vi "Main.vi"(11 "Module Admin":refnum<class "Delacor_lib_QMH_Cloneable Module Admin.lvclass">) -> ()   [LabVIEW 2016, in "Data Analysis.lvlib"]
doc: "This template is based off of the Queued Message Handler design pattern and the Queued Message Handler project template that ships with LabVIEW.\n\nThe main difference is that the queue is private to this module and communication between modules is performed via Broadcast and Request events.\n\nRequest events are wrapped in public API methods and are handled in the Event Handling Loop (EHL) of this VI. Any module can register for Broadcast events sent by this module. The EHL generates messages based on user interface actions.\n\nThe Message Handling Loop (MHL) processes messages generated by the EHL, or by other messages. The messages are string values, so new messages can be added easily to the Message Cases case structure in the MHL. Each message cluster can also provide an optional value for Message Data, which is a variant that can be converted to whatever message-specific data is required.\n_____\nBased on DQMH Project Template 6.1.0.94."
uses:
  Data Analysis.lvlib
  <vilib>/Delacor/Delacor QMH/Libraries/Cloneable Module Admin_class/Delacor_lib_QMH_Cloneable Module Admin.lvclass
  C:/Program Files (x86)/National Instruments/LabVIEW 2016/vi.lib/Delacor/Delacor QMH/Libraries/Module Admin_class/Delacor_lib_QMH_Module Admin.lvclass
  <vilib>/Delacor/Delacor QMH/Libraries/Cloneable Module Admin_class/Delacor_lib_QMH_Cloneable Module Admin.lvclass/Delacor_lib_QMH_Cloneable Module Admin.ctl
  Module Data--cluster.ctl
  <vilib>/Delacor/Delacor QMH/Libraries/Message Queue_class/Delacor_lib_QMH_Message Queue.lvclass/Delacor_lib_QMH_Message Queue.ctl
  Stop Argument--cluster.ctl
  REQ Initialize Selector Argument--cluster.ctl
  REQ Start Acq Argument--cluster.ctl
  REQ Signal Selection Argument--cluster.ctl
  REQ Stop Acq Argument--cluster.ctl
  <vilib>/Utility/miscctls.llb/LVPointTypeDef.ctl
  <vilib>/Delacor/Delacor QMH/Libraries/Module Admin_class/Delacor_lib_QMH_Module Admin.lvclass/Delacor_lib_QMH_Module Admin.ctl
  <vilib>/Delacor/Delacor QMH/Libraries/Cloneable Module Admin_class/Delacor_lib_QMH_Get Module ID.vi
  <vilib>/Delacor/Delacor QMH/Libraries/Message Queue_class/Delacor_lib_QMH_Enqueue Message (Single).vi
  Support Libraries/Current Value Table/DataTypes/Array of Double_Read.vi
  Support Libraries/Current Value Table/DataTypes/Double_Read.vi
  Support Libraries/Current Value Table/DataTypes/Single_Read.vi
  Support Libraries/Current Value Table/DataTypes/Boolean_Read.vi
  <vilib>/Delacor/Delacor QMH/Libraries/Module Admin_class/Delacor_lib_QMH_Get External Launch.vi
  Support Libraries/Current Value Table/Type to Enum.vi
  Support Libraries/Current Value Table/DataTypes/Array of Double_Type To Enum.vi
  Support Libraries/Current Value Table/DataTypes/Double_Type To Enum.vi
  Support Libraries/Current Value Table/DataTypes/Single_Type To Enum.vi
  Support Libraries/Current Value Table/DataTypes/Boolean_Type To Enum.vi
  <vilib>/Utility/error.llb/Error Cluster From Error Code.vi
  Support Libraries/Current Value Table/FGVs/Tag Memory.vi
  Support Libraries/Current Value Table/FGVs/CVT Globals.vi
  Support Libraries/Current Value Table/Memory Block.vi
  Support Libraries/Current Value Table/DataTypes/Array of Double_Memory Block.vi
  Support Libraries/Current Value Table/DataTypes/Double_Memory Block.vi
  Support Libraries/Current Value Table/DataTypes/Single_Memory Block.vi
  Support Libraries/Current Value Table/DataTypes/Boolean_Memory Block.vi
  <vilib>/ErrorRing/Error Ring.xnode
  <vilib>/Delacor/Delacor QMH/Libraries/Message Queue_class/Delacor_lib_QMH_Message Queue.lvclass
  User Interface/User Interface.lvlib
  Error Log/Error Log.lvlib
  Support Libraries/Current Value Table/Current Value Table.lvlib
panel:
  in  "Select Module":i32(ring)=-1 items=["All"=-1]
  in  "error in (no error)":errorcluster
  in  "Signal Selection":string[](tree)
  in  "Stop Button":bool
  in  "Start Button":bool
  out "Time":string="Sat  8/3/2019  8:10:44 PM"
  in  "Exit":bool
  out "Analog Data":dbl[][](graph)
  out "error out":errorcluster
  out "Status":string
  in  "Simulate EHL Error":bool
  in  "Simulate MHL Error":bool
  # "Other QMH Modules communicate with this Module via its Public API (wrappers for its Request Events).\n\nThis Module communicates with other Modules via its Broadcast Events.\nAny module that wants to get these messages, just registers for this module's Broadcast events."
  # "This template is for the Delacor Modified Queued Message Handler design pattern.\n\nSee the block diagram for more information on how to use this template."
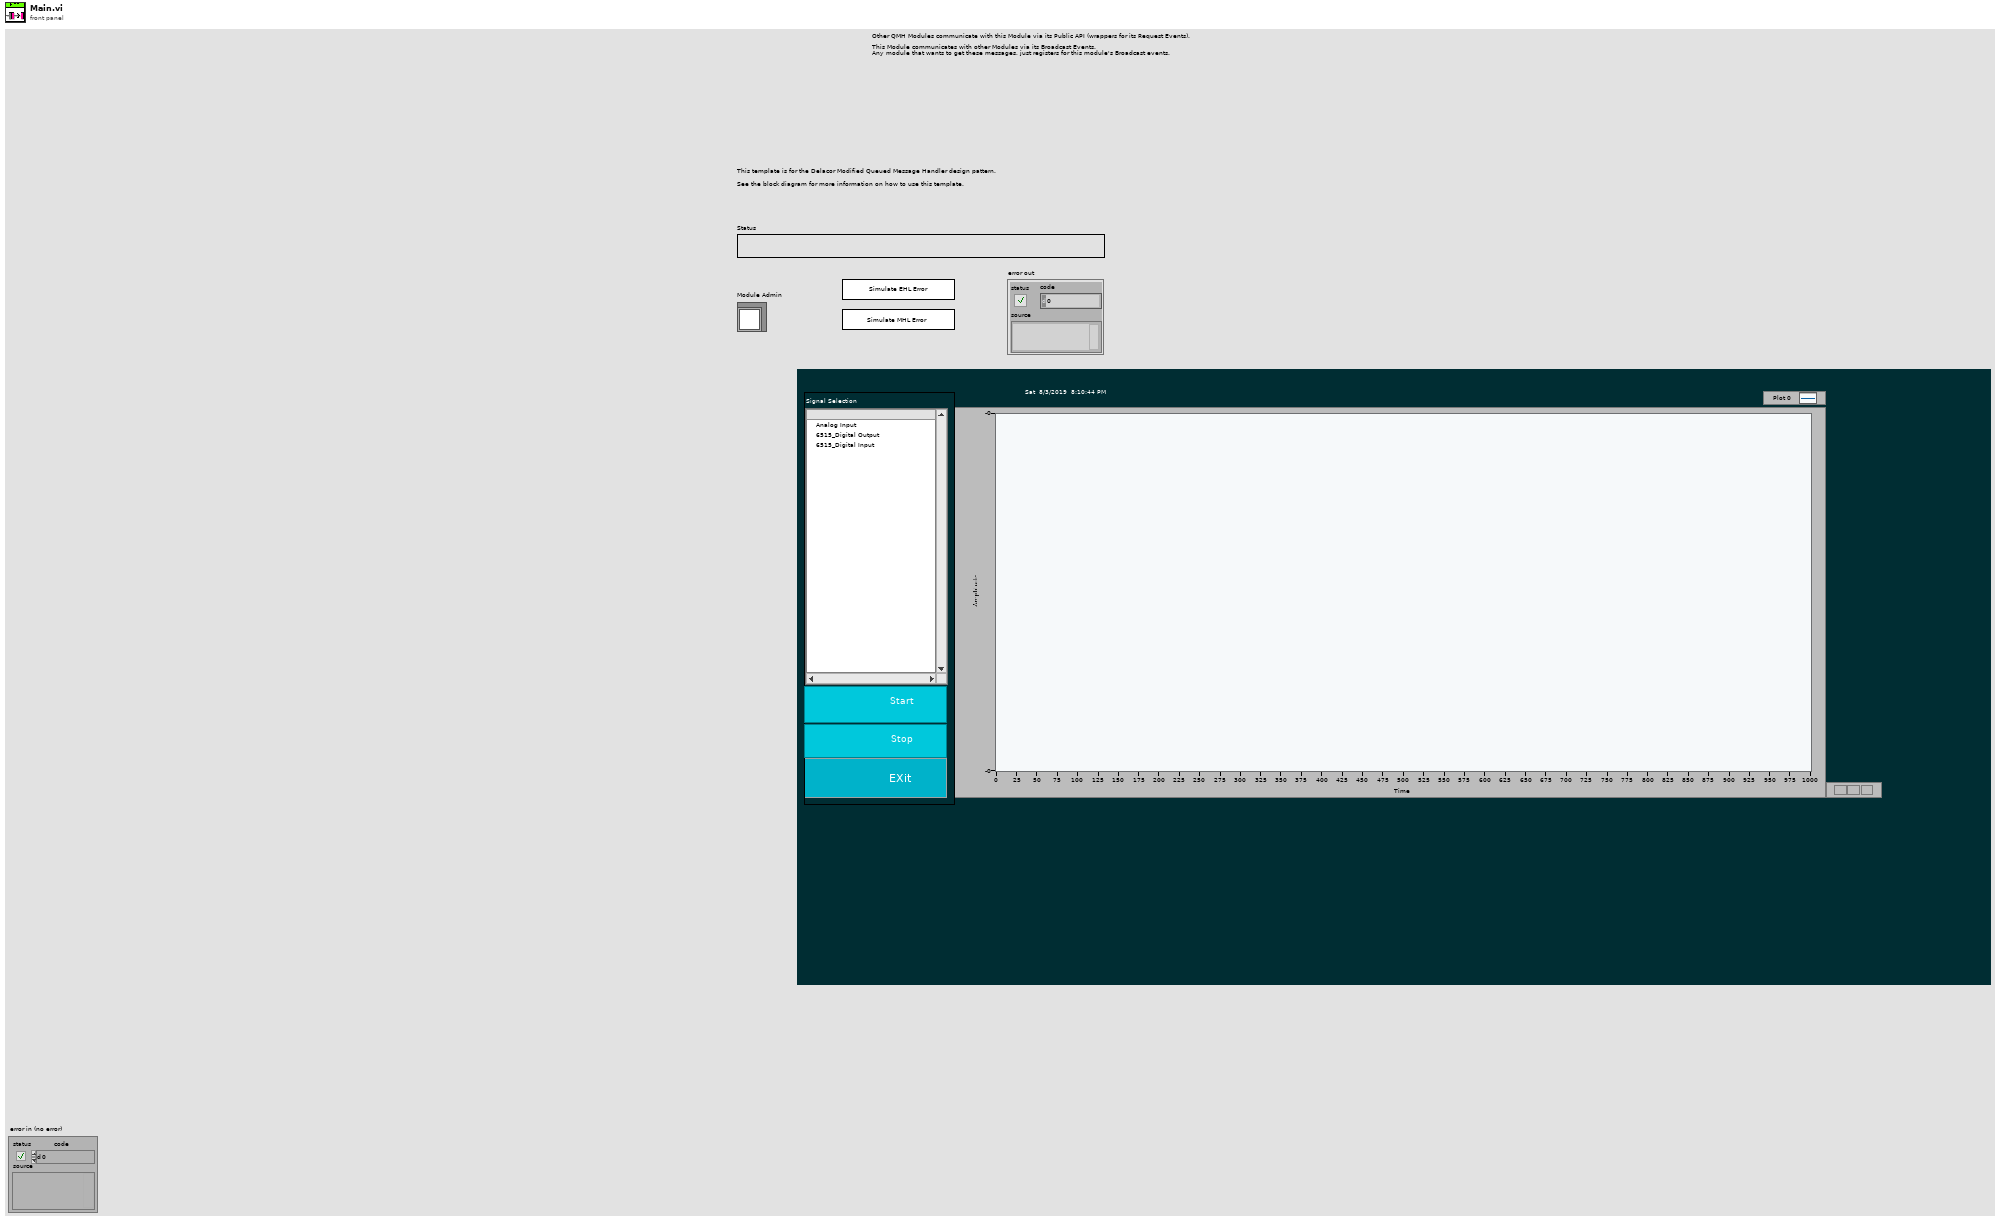
[diagram p1: front panel]
types:
  T1 = typedef "Data Analysis.lvlib/Request Events--cluster.ctl" = cluster{"Stop Module":refnum<user-event>, "Show Panel":refnum<user-event>, "Hide Panel":refnum<user-event>, "Show Diagram":refnum<user-event>, "Get Module Execution Status":refnum<user-event>, "REQ Initialize Selector":refnum<user-event>, "REQ Wakeup_help_loop":refnum<user-event>, "REQ Start Acq":refnum<user-event>, "REQ Signal Selection":refnum<user-event>, "REQ Stop Acq":refnum<user-event>}
  T2 = enum32{"invalid lock state", "Not Locked", "Locked (No Password)", "Password-protected"}
  T3 = typedef "Data Analysis.lvlib/Stop Argument--cluster.ctl" = cluster{"Module ID":i32, "Origin":string, "Exit via Stop Module Req?":bool, "Wait for Module to stop?":bool}
  T4 = typedef "Data Analysis.lvlib/REQ Initialize Selector Argument--cluster.ctl" = cluster{"Module ID":i32, "Boolean":bool}
  T5 = typedef "Data Analysis.lvlib/REQ Start Acq Argument--cluster.ctl" = cluster{"Module ID":i32, "Boolean":bool}
  T6 = typedef "Data Analysis.lvlib/REQ Signal Selection Argument--cluster.ctl" = cluster{"Module ID":i32, "Signal Selection":string[]}
  T7 = typedef "Data Analysis.lvlib/REQ Stop Acq Argument--cluster.ctl" = cluster{"Module ID":i32, "Boolean":bool}
  T8 = typedef "LVPointTypeDef.ctl" = cluster{"Horizontal":i16, "Vertical":i16}
  T9 = enum32{"Invalid", "Standard", "Closed", "Hidden", "Minimized", "Maximized"}
  T10 = typedef "Data Analysis.lvlib/Module Data--cluster.ctl" = cluster{"Status":string, "Signal Selecton":refnum<vi>, "Active Signal":string[], "Module ID":i32}
  T11 = typedef "CVT.lvlib/Current Value Table.lvlib/Data Types.ctl" = enum16{"Double", "Single", "I64", "I32", "I16", "I8", "U64", "U32", "U16", "U8", "String", "Boolean", "Array of U8", "Array of U16", "Array of U32", "Array of U64", "Array of I64", "Array of I32", "Array of I16", "Array of I8", "Array of Double", "Array of Single", "Array of Boolean", "Array of String"}
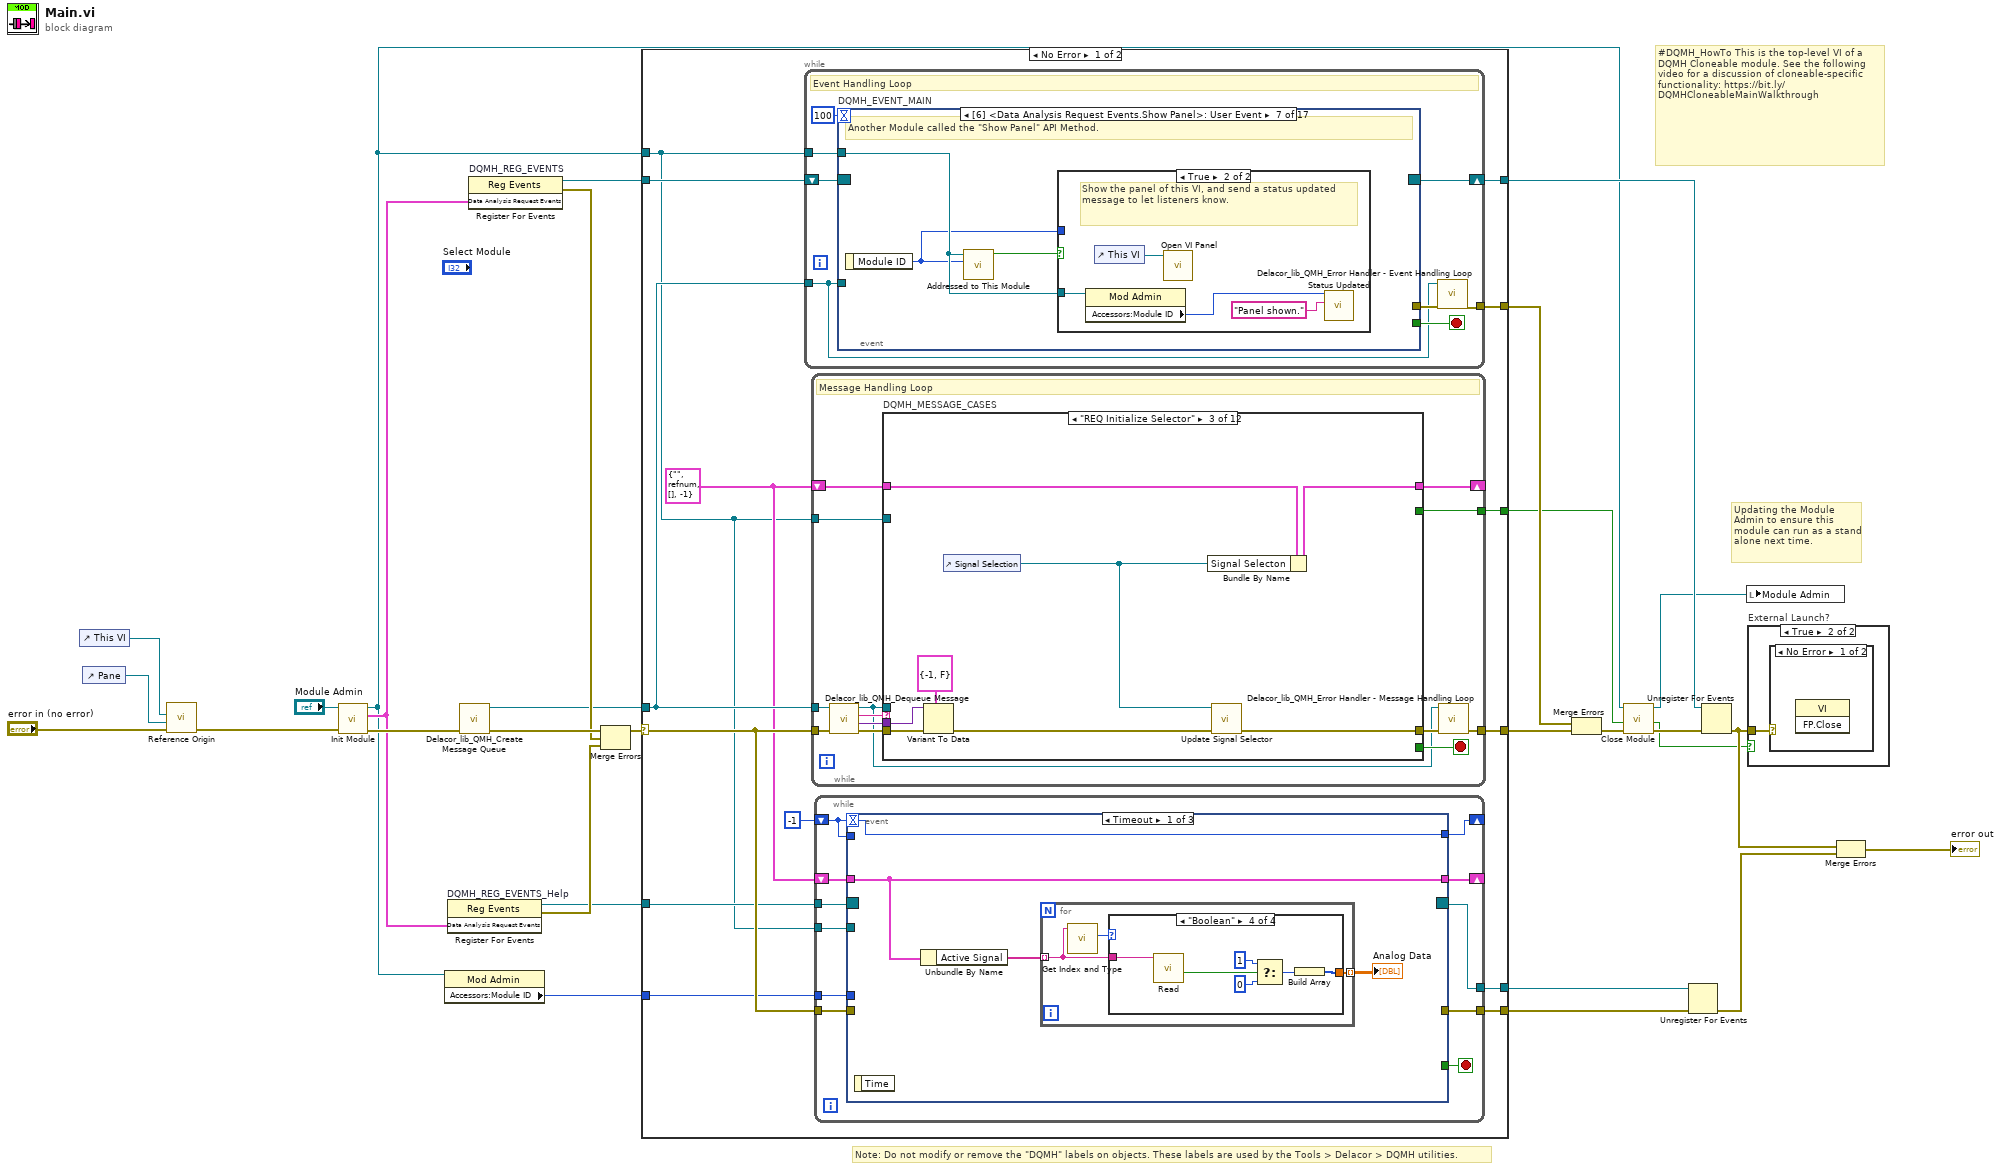
[diagram p0: block diagram]
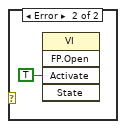
[diagram p3: hidden frame]
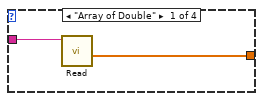
[diagram p4: hidden frame]
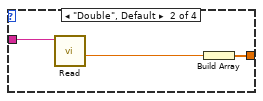
[diagram p5: hidden frame]
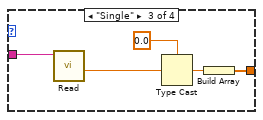
[diagram p6: hidden frame]
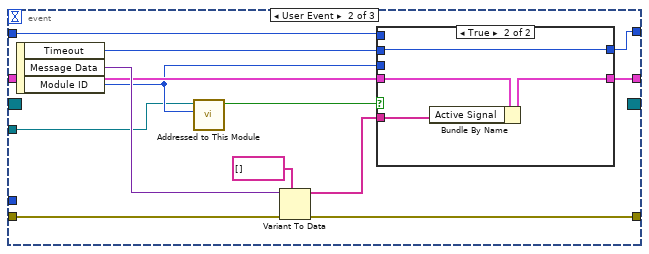
[diagram p7: hidden frame]
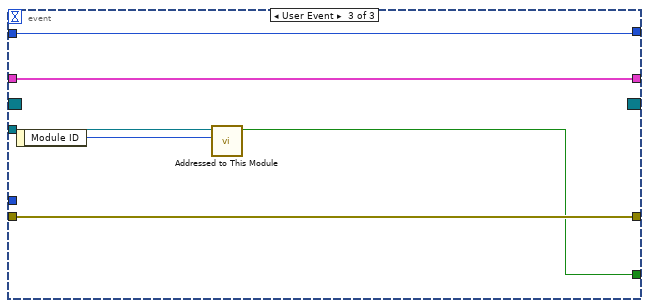
[diagram p9: hidden frame]
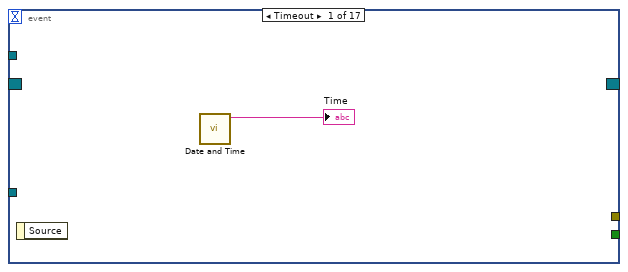
[diagram p10: hidden frame]
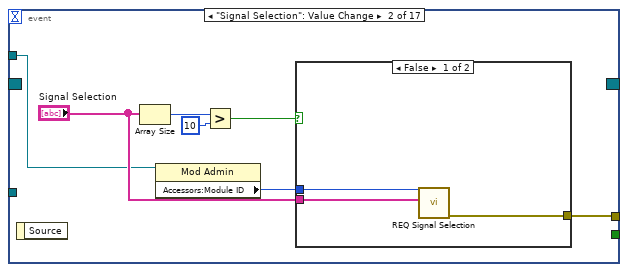
[diagram p11: hidden frame]
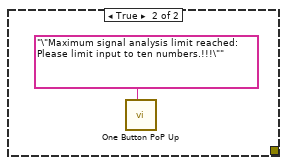
[diagram p12: hidden frame]
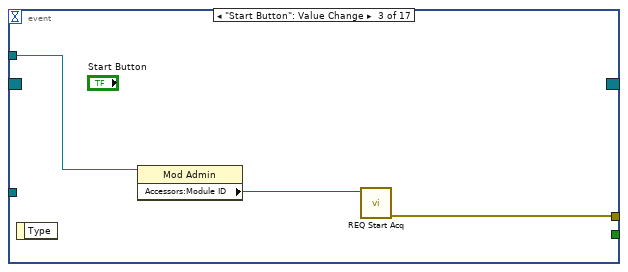
[diagram p13: hidden frame]
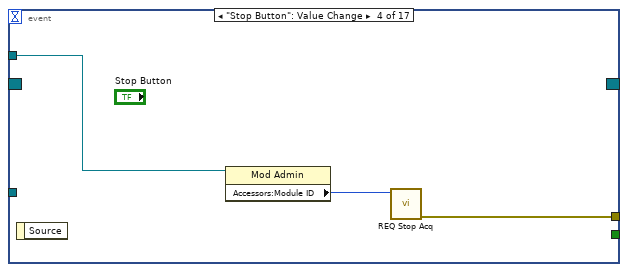
[diagram p14: hidden frame]
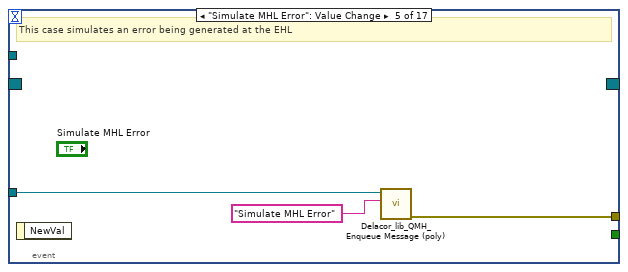
[diagram p15: hidden frame]
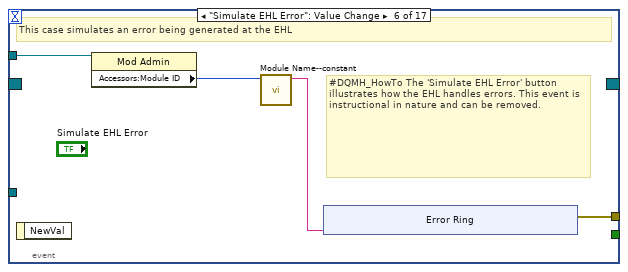
[diagram p16: hidden frame]
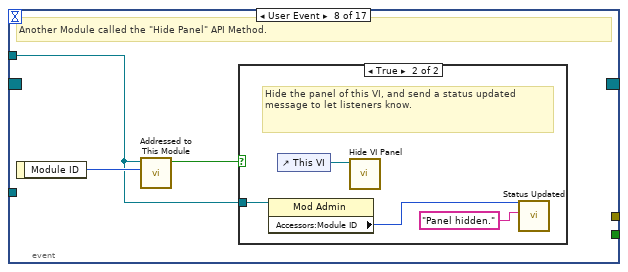
[diagram p18: hidden frame]
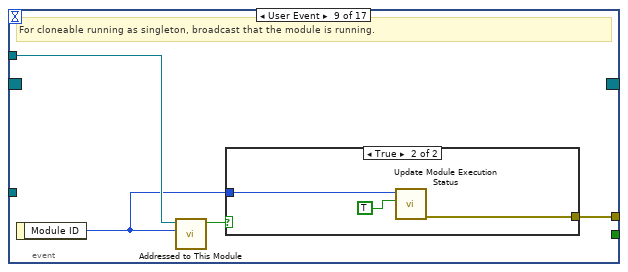
[diagram p20: hidden frame]
diagram:
  # "#DQMH_HowTo This is the top-level VI of a DQMH Cloneable module. See the following video for a discussion of cloneable-specific functionality: https://bit.ly/DQMHCloneableMainWalkthrough"
  # "Note: Do not modify or remove the \"DQMH\" labels on objects. These labels are used by the Tools > Delacor > DQMH utilities."
  # "Updating the Module Admin to ensure this module can run as a stand alone next time."
  n1 = control-ref of="This VI"() -> (w2:refnum<vi>)
  n2 = control-ref of="Pane"() -> (w1:refnum<vi>)
  n3 = call "Reference Origin.vi"("error in (no error)"="error in (no error)", "Pane"=w1, "This VI"=w2) -> ("error out"=w3:errorcluster)  [unwired: 8 in]
  n4 = call "Init Module.vi"("error in"=w3, "Cloneable Module Admin in"="Module Admin") -> ("error out"=w26:errorcluster, "Data Analysis Request Events"=w12:T1, "Cloneable Module Admin out"=w5:refnum<class "Delacor_lib_QMH_Cloneable Module Admin.lvclass">)  [unwired: 7 in]
  n5 = property class="Mod Admin"(reference=w5) -> ("Accessors:Module ID"=w4:i32)  [unwired: 1 in, 2 out]
  n6 = register-events "DQMH_REG_EVENTS_Help"(w12) -> (reference out=w10:refnum<event-registration>, error out=w11:errorcluster)  [unwired: 2 in]
  n7 = call <vilib>:"Delacor_lib_QMH_Create Message Queue.vi"("error in"=w26) -> ("error out"=w23:errorcluster, "Message Queue"=w18:refnum<class "Delacor_lib_QMH_Message Queue.lvclass">)  [unwired: 9 in]
  n8 = register-events "DQMH_REG_EVENTS"(w12) -> (reference out=w19:refnum<event-registration>, error out=w21:errorcluster)  [unwired: 2 in]
  n9 = Merge Errors(w23, w21, w11) -> (w22:errorcluster)
  n10 = case shown="No Error" w22 {
    selector: w22 -> [w37 w403]
    tunnel: [w43 w402] -> w27
    tunnel: [w41 w410] -> w20
    tunnel: w19 -> [w40 w410]
    tunnel: w18 -> [w39 w401]
    tunnel: [w42 _] -> w28
    tunnel: w5 -> [w30 w406]
    tunnel: [w38 _] -> w15
    tunnel: w10 -> [w36 w400]
    tunnel: [w35 _] -> w9
    tunnel: [w34 w400] -> w8
    tunnel: w4 -> [w31 _]
    frame No Error {
      w33 = T10 {"Status"="", "Signal Selecton"=refnum, "Active Signal"=[], "Module ID"=-1} ("Data Cluster")
      n11 = while {
        tunnel: w39 -> [w104]
        shift-right: [w107] -> w41
        shift-left: w40 -> [w108]
        tunnel: [w109] -> w42
        tunnel: w30 -> [w105]
        stop <- w106 stop-if-true
        # "Event Handling Loop"
        n12 = event "DQMH_EVENT_MAIN" shown="[6] <Data Analysis Request Events.Show Panel>: User Event" {
          selector: w108 -> [_ _ _ _ _ _ _ _ _ _ _ _ _ _ _ _ _]
          dyn-events: [_ _ _ _ _ _ _ _ _ _ _ _ _ _ _ _ _] -> w107
          timeout: 100 -> [_ _ _ _ _ _ _ _ _ _ _ _ _ _ _ _ _]
          tunnel: [_ _ _ _ _ _ _ _ _ _ w183 _ _ _ _ _ _] -> w106
          tunnel: w104 -> [_ _ _ _ w130 _ _ _ _ _ w186 w203 w209 w217 w229 w241 w253]
          tunnel: [_ w114 w125 w128 w131 w135 _ _ w160 _ w187 w205 w208 w210 w222 w234 w246] -> w110
          tunnel: w105 -> [_ w113 w124 w127 _ w134 w144 w150 w158 w164 w185 _ _ w215 w227 w239 w251]
          event Timeout {
            n13 = event-data() -> ()  [unwired: 1 in, 1 out]
            n14 = call "Date and Time.vi"() -> ("Current Time"=→"Time":string)  [unwired: 11 in]
          }
          event "Signal Selection": Value Change {
            n15 = event-data() -> ()  [unwired: 1 in, 1 out]
            n16 = Array Size(array="Signal Selection") -> (size(s)=w118:i32)
            n17 = property class="Mod Admin"(reference=w113) -> ("Accessors:Module ID"=w112:i32)  [unwired: 1 in, 2 out]
            n18 = Greater?(x=w118, y=10) -> (0:w116:bool)
            n19 = case shown="False" w116 {
              tunnel: "Signal Selection" -> [w120 _]
              tunnel: [w121 _] -> w114
              tunnel: w112 -> [w119 _]
              frame False {
                n20 = call "REQ Signal Selection.vi"("Signal Selection"=w120, "Module ID"=w119) -> ("error out"=w121:errorcluster)  [unwired: 9 in]
              }
              frame True {
                n21 = call "One Button PoP Up.vi"("Message In"="\"Maximum signal analysis limit reached: Please limit input to ten numbers.!!!\"") -> ()  [unwired: 11 in]
              }
            }
          }
          event "Start Button": Value Change {
            n22 = event-data() -> ()  [unwired: 1 in, 1 out]
            n23 = property class="Mod Admin"(reference=w124) -> ("Accessors:Module ID"=w123:i32)  [unwired: 1 in, 2 out]
            n24 = call "REQ Start Acq.vi"("Module ID"=w123) -> ("error out"=w125:errorcluster)  [unwired: 10 in]
          }
          event "Stop Button": Value Change {
            n25 = event-data() -> ()  [unwired: 1 in, 1 out]
            n26 = property class="Mod Admin"(reference=w127) -> ("Accessors:Module ID"=w126:i32)  [unwired: 1 in, 2 out]
            n27 = call "REQ Stop Acq.vi"("Module ID"=w126) -> ("error out"=w128:errorcluster)  [unwired: 10 in]
          }
          event "Simulate MHL Error": Value Change {
            # "This case simulates an error being generated at the EHL"
            n28 = event-data() -> ()  [unwired: 1 in, 1 out]
            n29 = call-poly <vilib>:"Delacor_lib_QMH_Enqueue Message (poly).vi"("Message"="Simulate MHL Error", "Message Queue in"=w130) -> ("error out"=w131:errorcluster)  [unwired: 8 in, 1 out]
          }
          event "Simulate EHL Error": Value Change {
            # "#DQMH_HowTo The 'Simulate EHL Error' button  illustrates how the EHL handles errors. This event is instructional in nature and can be removed."
            # "This case simulates an error being generated at the EHL"
            n30 = event-data() -> ()  [unwired: 1 in, 1 out]
            n31 = property class="Mod Admin"(reference=w134) -> ("Accessors:Module ID"=w133:i32)  [unwired: 1 in, 2 out]
            n32 = call "Module Name--constant.vi"("Module ID"=w133) -> ("Module Name"=w132:string)  [unwired: 10 in]
            n33 = xnode "Error Ring"("parameter 0"=w132) -> ("error out"=w135:errorcluster)
          }
          event User Event {
            # "Another Module called the \"Show Panel\" API Method."
            n34 = event-data() -> ("Module ID"=w143:i32)  [unwired: 1 in]
            n35 = call "Addressed to This Module.vi"("Module ID from Argument"=w143, "Module Admin"=w144) -> ("Addressed to this instance?"=w145:bool)  [unwired: 8 in, 1 out]
            n36 = case shown="True" w145 {
              tunnel: w144 -> [_ w147]
              tunnel: w143 -> [_ _]
              frame False {
              }
              frame True {
                # "Show the panel of this VI, and send a status updated message to let listeners know."
                n37 = property class="Mod Admin"(reference=w147) -> ("Accessors:Module ID"=w146:i32)  [unwired: 1 in, 2 out]
                n38 = control-ref of="This VI"() -> (w149:refnum<vi>)
                n39 = call "Open VI Panel.vi"("VI"=w149) -> ()  [unwired: 10 in, 1 out]
                n40 = call "Status Updated.vi"("Status"="Panel shown." ("format string"), "Module ID"=w146) -> ()  [unwired: 9 in, 1 out]
              }
            }
          }
          event User Event {
            # "Another Module called the \"Hide Panel\" API Method."
            n41 = event-data() -> ("Module ID"=w151:i32)  [unwired: 1 in]
            n42 = call "Addressed to This Module.vi"("Module ID from Argument"=w151, "Module Admin"=w150) -> ("Addressed to this instance?"=w152:bool)  [unwired: 8 in, 1 out]
            n43 = case shown="True" w152 {
              tunnel: w150 -> [_ w154]
              frame False {
              }
              frame True {
                # "Hide the panel of this VI, and send a status updated message to let listeners know."
                n44 = property class="Mod Admin"(reference=w154) -> ("Accessors:Module ID"=w153:i32)  [unwired: 1 in, 2 out]
                n45 = control-ref of="This VI"() -> (w156:refnum<vi>)
                n46 = call "Hide VI Panel.vi"("VI"=w156) -> ()  [unwired: 10 in, 1 out]
                n47 = call "Status Updated.vi"("Status"="Panel hidden." ("format string"), "Module ID"=w153) -> ()  [unwired: 9 in, 1 out]
              }
            }
          }
          event User Event {
            # "For cloneable running as singleton, broadcast that the module is running."
            n48 = event-data() -> ("Module ID"=w157:i32)  [unwired: 1 in]
            n49 = call "Addressed to This Module.vi"("Module ID from Argument"=w157, "Module Admin"=w158) -> ("Addressed to this instance?"=w159:bool)  [unwired: 8 in, 1 out]
            n50 = case shown="True" w159 {
              tunnel: [_ w163] -> w160
              tunnel: w157 -> [_ w162]
              frame False {
              }
              frame True {
                n51 = call "Update Module Execution Status.vi"("Running?"=TRUE, "Module ID"=w162) -> ("error out"=w163:errorcluster)  [unwired: 9 in]
              }
            }
          }
          event User Event {
            # "Another Module called the \"Show Diagram\" API Method. This event is used for debugging."
            n52 = event-data() -> ("Module ID"=w165:i32)  [unwired: 1 in]
            n53 = call "Addressed to This Module.vi"("Module ID from Argument"=w165, "Module Admin"=w164) -> ("Addressed to this instance?"=w166:bool)  [unwired: 8 in, 1 out]
            n54 = case shown="True" w166 {
              tunnel: w164 -> [_ w167]
              frame False {
              }
              frame True {
                n55 = disable-structure shown="RUN_TIME_ENGINE==False" {
                  disable-tunnel: w167 -> [w168 _]
                  frame condition #0 (active) {
                    # "functionality not available in exe"
                    n56 = invoke class="VI" method="Lock State.Get"() -> (error out=w174:errorcluster, "Get Lock State"=w173:T2, "pwd in cache"=w170:bool)  [unwired: 4 in, 1 out]
                    n57 = Equal?(x=T2."Password-protected", y=w173) -> (x = y?=w171:bool)
                    n58 = Compound Arithmetic op=AND(w171, invert w170) -> (w169:bool)
                    n59 = case shown="False" w169 {
                      tunnel: w174 -> [w179 _]
                      tunnel: w168 -> [w176 _]
                      frame False {
                        n60 = property class="Mod Admin"(reference=w176) -> ("Accessors:Module ID"=w175:i32)  [unwired: 1 in, 2 out]
                        n61 = property class="VI"(error in=w179, "BDWin.Open"=TRUE ("Block Diagram Window:Open")) -> ()  [unwired: 1 in, 2 out]
                        n62 = call "Status Updated.vi"("Status"="Block Diagram shown." ("format string"), "Module ID"=w175) -> ()  [unwired: 9 in, 1 out]
                      }
                      frame True {
                        # "Password-protected VI, and the password is not in the cache. Do not show the diagram."
                      }
                    }
                  }
                  frame condition #1 {
                  }
                }
              }
            }
          }
          event User Event {
            # "Another Module called the \"Stop Module\" API Method  or the Message Handling Loop below."
            n63 = event-data() -> ("Module ID"=w181:i32, "Wait for Module to stop?"=w182:bool, "Origin"=w180:string)  [unwired: 1 in]
            n64 = call "Addressed to This Module.vi"("Module ID from Argument"=w181, "Module Admin"=w185) -> ("Addressed to this instance?"=w184:bool)  [unwired: 8 in, 1 out]
            n65 = case shown="True" w184 {
              tunnel: [_ w199] -> w187
              tunnel: w186 -> [_ w195]
              tunnel: [_ TRUE] -> w183
              tunnel: w182 -> [_ w190]
              tunnel: w181 -> [_ w192]
              tunnel: w180 -> [_ w188]
              frame False {
              }
              frame True {
                # "The event can get fired from the Exit message. The queue gets destroyed there. In this case, the Enqueue VI will return error 1. It is safe to ignore, because the module is already exiting."
                n66 = local write "Status"(w188) -> ()
                n67 = Bundle By Name(cluster=T3 {"Module ID"=-1, "Origin"="", "Exit via Stop Module Req?"=FALSE, "Wait for Module to stop?"=FALSE} ("Stop Argument"), "Module ID"=w192, "Exit via Stop Module Req?"=TRUE, "Wait for Module to stop?"=w190) -> (w189:T3)
                n68 = call-poly <vilib>:"Delacor_lib_QMH_Enqueue Message (poly).vi"("Priority Message? (F)"=TRUE, "Message Data"=w189, "Message"="Exit", "Message Queue in"=w195) -> ("error out"=w200:errorcluster)  [unwired: 6 in, 1 out]
                n69 = call <vilib>:"Clear Errors.vi"("error in (no error)"=w200, "specific error code to clear (0: all)"=1) -> ("error out"=w199:errorcluster)  [unwired: 4 in, 1 out]
              }
            }
          }
          event Panel Close? {
            w204 = TRUE  # Discard the event, the MHL is responsible for closing and stopping this VI.
            # "Hide the panel or send the 'Exit' message if the user clicks the 'X' on the module main VI panel."
            n70 = event-data() -> ()  [unwired: 1 in, 1 out]
            n71 = call-poly <vilib>:"Delacor_lib_QMH_Enqueue Message (poly).vi"("Priority Message? (F)"=TRUE, "Message"="Exit", "Message Queue in"=w203) -> ("error out"=w205:errorcluster)  [unwired: 7 in, 1 out]
            n72 = event-data("Discard?"=w204) -> ()  [unwired: 1 in, 1 out]
          }
          event "Exit": Value Change {
            n73 = event-data() -> ()  [unwired: 1 in, 1 out]
            n74 = call-poly <vilib>:"Delacor_lib_QMH_Enqueue Message (poly).vi"("Priority Message? (F)"=TRUE, "Message"="Exit", "Message Queue in"=w209) -> ("error out"=w208:errorcluster)  [unwired: 7 in, 1 out]
          }
          event User Event {
            # "Another Module called the \"REQ Initialize Selector\" API Method."
            n75 = event-data() -> ("Module ID"=w212:i32, "Boolean"=w211:bool)  [unwired: 1 in]
            n76 = Bundle(cluster=T4 {"Module ID"=-1, "Boolean"=FALSE} ("REQ Initialize Selector Argument"), "Module ID"=w212, "Boolean"=w211) -> (w213:T4)
            n77 = call "Addressed to This Module.vi"("Module ID from Argument"=w212, "Module Admin"=w215) -> ("Addressed to this instance?"=w216:bool)  [unwired: 8 in, 1 out]
            n78 = case shown="True" w216 {
              tunnel: w217 -> [_ w221]
              tunnel: w213 -> [_ w219]
              tunnel: [_ w218] -> w210
              frame False {
              }
              frame True {
                n79 = call-poly <vilib>:"Delacor_lib_QMH_Enqueue Message (poly).vi"("Message Data"=w219, "Message"="REQ Initialize Selector", "Message Queue in"=w221) -> ("error out"=w218:errorcluster)  [unwired: 7 in, 1 out]
              }
            }
          }
          event User Event {
            # "Another Module called the \"REQ Start Acq\" API Method."
            n80 = event-data() -> ("Module ID"=w224:i32, "Boolean"=w223:bool)  [unwired: 1 in]
            n81 = Bundle(cluster=T5 {"Module ID"=-1, "Boolean"=FALSE} ("REQ Start Acq Argument"), "Module ID"=w224, "Boolean"=w223) -> (w225:T5)
            n82 = call "Addressed to This Module.vi"("Module ID from Argument"=w224, "Module Admin"=w227) -> ("Addressed to this instance?"=w228:bool)  [unwired: 8 in, 1 out]
            n83 = case shown="True" w228 {
              tunnel: w229 -> [_ w233]
              tunnel: w225 -> [_ w231]
              tunnel: [_ w230] -> w222
              frame False {
              }
              frame True {
                n84 = call-poly <vilib>:"Delacor_lib_QMH_Enqueue Message (poly).vi"("Message Data"=w231, "Message"="REQ Start Acq", "Message Queue in"=w233) -> ("error out"=w230:errorcluster)  [unwired: 7 in, 1 out]
              }
            }
          }
          event User Event {
            # "Another Module called the \"REQ Signal Selection\" API Method."
            n85 = event-data() -> ("Module ID"=w236:i32, "Signal Selection"=w235:string[])  [unwired: 1 in]
            n86 = Bundle(cluster=T6 {"Module ID"=-1, "Signal Selection"=[]} ("REQ Signal Selection Argument"), "Module ID"=w236, "Signal Selection"=w235) -> (w237:T6)
            n87 = call "Addressed to This Module.vi"("Module ID from Argument"=w236, "Module Admin"=w239) -> ("Addressed to this instance?"=w240:bool)  [unwired: 8 in, 1 out]
            n88 = case shown="True" w240 {
              tunnel: w241 -> [_ w245]
              tunnel: w237 -> [_ w243]
              tunnel: [_ w242] -> w234
              frame False {
              }
              frame True {
                n89 = call-poly <vilib>:"Delacor_lib_QMH_Enqueue Message (poly).vi"("Message Data"=w243, "Message"="REQ Signal Selection", "Message Queue in"=w245) -> ("error out"=w242:errorcluster)  [unwired: 7 in, 1 out]
              }
            }
          }
          event User Event {
            # "Another Module called the \"REQ Stop Acq\" API Method."
            n90 = event-data() -> ("Module ID"=w248:i32, "Boolean"=w247:bool)  [unwired: 1 in]
            n91 = Bundle(cluster=T7 {"Module ID"=-1, "Boolean"=FALSE} ("REQ Stop Acq Argument"), "Module ID"=w248, "Boolean"=w247) -> (w249:T7)
            n92 = call "Addressed to This Module.vi"("Module ID from Argument"=w248, "Module Admin"=w251) -> ("Addressed to this instance?"=w252:bool)  [unwired: 8 in, 1 out]
            n93 = case shown="True" w252 {
              tunnel: w253 -> [_ w257]
              tunnel: w249 -> [_ w255]
              tunnel: [_ w254] -> w246
              frame False {
              }
              frame True {
                n94 = call-poly <vilib>:"Delacor_lib_QMH_Enqueue Message (poly).vi"("Message Data"=w255, "Message"="REQ Stop Acq", "Message Queue in"=w257) -> ("error out"=w254:errorcluster)  [unwired: 7 in, 1 out]
              }
            }
          }
        }
        n95 = call-dynamic "Delacor_lib_QMH_Error Handler - Event Handling Loop.vi"("error in"=w110, "Message Queue in"=w104) -> ("dup error in"=w109:errorcluster)  [unwired: 8 in, 1 out]
      }
      n96 = while {
        tunnel: w39 -> [w261]
        shift-right: [w265] -> _
        shift-left: w33 -> [w266]
        tunnel: w37 -> [w269]
        tunnel: [w267] -> w43
        tunnel: w30 -> [w259]
        tunnel: [w258] -> w38
        stop <- w264 stop-if-true
        # "Message Handling Loop"
        n97 = call-dynamic "Delacor_lib_QMH_Dequeue Message.vi"("error in"=w269, "Message Queue in"=w261) -> ("error out"=w268:errorcluster, "Message Data"=w262:variant, "Message"=w263:string, "Message Queue out"=w260:refnum<class "Delacor_lib_QMH_Message Queue.lvclass">)  [unwired: 6 in]
        n98 = case "DQMH_MESSAGE_CASES" shown="\"REQ Initialize Selector\"" w263 {
          selector: w263 -> [_ _ _ _ _ _ _ _ _ _ _ w387]
          tunnel: w260 -> [_ _ _ _ _ _ _ _ w339 _ w368 _]
          tunnel: w268 -> [w289 w293 w301 w312 w320 w331 w334 w336 w348 w360 w383 w389]
          tunnel: [w271 w293 w296 w304 w318 w322 w333 w336 w344 w359 w380 w390] -> w270
          tunnel: w266 -> [w281 w292 w300 w306 w319 w325 w332 w335 w343 w357 w377 w388]
          tunnel: [w280 w292 w295 w306 w314 w325 w332 w335 w343 w357 w377 w388] -> w265
          tunnel: [_ _ _ _ _ _ _ _ _ _ w376 _] -> w264
          tunnel: w262 -> [_ _ w299 w311 w317 w330 _ _ w342 _ w374 _]
          tunnel: w259 -> [w276 _ _ _ _ _ _ _ w341 w355 w370 w385]
          tunnel: [_ _ _ _ _ _ _ _ _ _ w372 _] -> w258
          frame "Initialize" {
            w273 = "Initial Message" ("Initial Message")
            # "Initialize - Any operation that needs to be done before the module can receive messages. Synchronize Caller Events.vi will inform Start Module.vi that the module has launched and is ready to receive messages. Module Did Init.vi will broadcast that the module initialized."
            n99 = call "Synchronize Caller Events.vi"("error in (no error)"=w289, "Module Admin"=w276) -> ("error out"=w288:errorcluster, "Module Admin out"=w275:refnum<class "Delacor_lib_QMH_Cloneable Module Admin.lvclass">)  [unwired: 8 in]
            n100 = property class="Mod Admin"(reference=w275) -> ("Accessors:Module ID"=w272:i32, "Accessors:External Launch"=w277:bool)  [unwired: 1 in, 2 out]
            n101 = call "Module Name--constant.vi"("Module ID"=w272) -> ("Module Name"=w285:string)  [unwired: 10 in]
            n102 = local write "Select Module"(w272) -> ()
            n103 = call "Module Name--constant.vi"("Module ID"=w272) -> ("Module Name"=w278:string)  [unwired: 10 in]
            n104 = call "Module Did Init.vi"("error in (no error)"=w288, "Initialized?"=TRUE, "Origin"=w278, "Module ID"=w272) -> ("error out"=w271:errorcluster)  [unwired: 7 in]
            n105 = property class="VI"("Front Panel.Title"=w285) -> (reference out=w287:refnum<vi>, error out=w291:errorcluster)  [unwired: 2 in]
            n106 = Select(t=T9."Hidden" ("State"), s=w277, f=T9."Standard" ("State")) -> (s? t:f=w282:T9)
            n107 = invoke class="VI" method="FP.Open"(reference=w287, error in=w291, "State"=w282) -> (reference out=w286:refnum<vi>, error out=w290:errorcluster)  [unwired: 2 in, 3 out]
            n108 = Bundle By Name(cluster=w281, "Status"=w273) -> (w280:T10)
            n109 = invoke class="VI" method="FP.Center"(reference=w286, error in=w290) -> ()  [unwired: 1 in, 3 out]
            n110 = property on="Pane" class="Pane"("Origin"=T8 {"Horizontal"=0, "Vertical"=0}) -> ()  [unwired: 2 in, 2 out]
            "Status" <- w273
          }
          frame "---Module Specific---" {
            # "Separator -- The following cases handle messages specific to this Module."
          }
          frame "REQ Initialize Selector" {
            n111 = Variant To Data(error in=w301, type=T4 {"Module ID"=-1, "Boolean"=FALSE} ("REQ Initialize Selector Argument"), Variant=w299) -> (error out=w297:errorcluster)  [unwired: 1 out]
            n112 = control-ref of="Signal Selection"() -> (w294:refnum<vi>)
            n113 = Bundle By Name(cluster=w300, "Signal Selecton"=w294) -> (w295:T10)
            n114 = call "Update Signal Selector.vi"("error in (no error)"=w297, "Signal Selecton"=w294) -> ("error out"=w296:errorcluster)  [unwired: 9 in]
          }
          frame "REQ Start Acq" {
            n115 = Variant To Data(error in=w312, type=T5 {"Module ID"=-1, "Boolean"=FALSE} ("REQ Start Acq Argument"), Variant=w311) -> (data=w309:T5, error out=w305:errorcluster)
            n116 = Unbundle By Name(w309) -> ("Module ID"=w302:i32)
            n117 = Unbundle By Name(w306) -> ("Active Signal"=w308:string[])
            n118 = To Variant(anything=w308) -> (Variant=w307:variant)
            n119 = call "REQ Wakeup_help_loop.vi"("error in"=w305, "Message Data"=w307, "Timeout"=0, "Module ID"=w302) -> ("error out"=w304:errorcluster)  [unwired: 7 in]
          }
          frame "REQ Signal Selection" {
            n120 = Variant To Data(error in=w320, type=T6 {"Module ID"=-1, "Signal Selection"=[]} ("REQ Signal Selection Argument"), Variant=w317) -> (data=w315:T6, error out=w318:errorcluster)
            n121 = Unbundle By Name(w315) -> ("Signal Selection"=w313:string[])
            n122 = Bundle By Name(cluster=w319, "Active Signal"=w313) -> (w314:T10)
          }
          frame "REQ Stop Acq" {
            n123 = Variant To Data(error in=w331, type=T7 {"Module ID"=-1, "Boolean"=FALSE} ("REQ Stop Acq Argument"), Variant=w330) -> (data=w328:T7, error out=w323:errorcluster)
            n124 = Unbundle By Name(w328) -> ("Module ID"=w321:i32)
            n125 = Unbundle By Name(w325) -> ("Active Signal"=w324:string[])
            n126 = To Variant(anything=w324) -> (Variant=w326:variant)
            n127 = call "REQ Wakeup_help_loop.vi"("error in"=w323, "Message Data"=w326, "Timeout"=-1, "Module ID"=w321) -> ("error out"=w322:errorcluster)  [unwired: 7 in]
          }
          frame "---Copy This Frame---" {
            # "Duplicate this frame when creating new messages.  Change this comment in the duplicated frame to describe this message."
            n128 = Merge Errors(w334) -> (w333:errorcluster)
          }
          frame "---Exit and Error Handling---" {
            # "Separator - the following cases handle errors and exit messages."
          }
          frame "Error" {
            # "Error - Check the error message data and respond accordingly. This message is sent by the \"Error Handler\" VIs at the end of each loop in this application."
            n129 = property class="Mod Admin"(reference=w341) -> ("Accessors:External Launch"=w340:bool, "Accessors:Module ID"=w338:i32)  [unwired: 1 in, 2 out]
            n130 = Variant To Data(error in=w348, type=errorcluster {"status"=FALSE, "code"=0, "source"=""} ("error constant"), Variant=w342) -> (data=w337:errorcluster, error out=w346:errorcluster)
            n131 = call "Error Reported.vi"("Error"=w337, "Module ID"=w338) -> ()  [unwired: 9 in, 1 out]
            n132 = call "REQ Log Error.vi"("error in (no error)"=w337) -> ()  [unwired: 10 in, 1 out]
            n133 = case shown="False" w340 {
              tunnel: [w353 _] -> w345
              tunnel: w339 -> [w351 _]
              tunnel: w337 -> [w352 _]
              frame False {
                # "If the module is running standalone, then pop up an error dialog and call the \"Exit\" message."
                n134 = call <vilib>:"Simple Error Handler.vi"("error in (no error)"=w352) -> ()  [unwired: 4 in, 5 out]
                n135 = call-poly <vilib>:"Delacor_lib_QMH_Enqueue Message (poly).vi"("Priority Message? (F)"=TRUE, "Message"="Exit", "Message Queue in"=w351) -> ("error out"=w353:errorcluster)  [unwired: 7 in, 1 out]
              }
              frame True {
                # "If the module was launched externally, calling the Error Reported broadcast VI is the only action performed by the \"Error\" message. The module's caller can then process the error appropriately."
              }
            }
            n136 = Merge Errors(w346, w345) -> (w344:errorcluster)
            n137 = local write "error out"(w344) -> ()
          }
          frame "Simulate MHL Error" {
            # "#DQMH_HowTo The 'Simulate MHL Error' button  illustrates how the MHL handles errors. This event is instructional in nature and can be removed."
            # "Simulate an error occurring at the MHL"
            n138 = property class="Mod Admin"(reference=w355) -> ("Accessors:Module ID"=w356:i32)  [unwired: 1 in, 2 out]
            n139 = call "Module Name--constant.vi"("Module ID"=w356) -> ("Module Name"=w354:string)  [unwired: 10 in]
            n140 = xnode "Error Ring"("parameter 0"=w354) -> ("error out"=w358:errorcluster)
            n141 = Merge Errors(w360, w358) -> (w359:errorcluster)
          }
          frame "Exit" {
            w375 = 91  # 91: not all Exit messages will have an argument
            w376 = TRUE  # Stop the VI
            # "Release the message queue reference"
            # "Exit - Exit the application."
            n142 = Variant To Data(error in=w383, type=T3 {"Module ID"=-1, "Origin"="", "Exit via Stop Module Req?"=FALSE, "Wait for Module to stop?"=FALSE} ("Stop Argument"), Variant=w374) -> (data=w371:T3, error out=w378:errorcluster)
            n143 = call <vilib>:"Clear Errors.vi"("error in (no error)"=w378, "specific error code to clear (0: all)"=w375) -> ("error out"=w382:errorcluster)  [unwired: 4 in, 1 out]
            n144 = control-ref of="This VI"() -> (w369:refnum<vi>)
            n145 = call "Handle Exit.vi"("Stop Argument"=w371, "Module Admin in"=w370, "VI reference"=w369) -> ("error out"=w379:errorcluster, "Wait for Stop?"=w372:bool)  [unwired: 7 in]
            n146 = call-dynamic "Delacor_lib_QMH_Release Message Queue.vi"("error in"=w382, "Message Queue"=w368) -> ("error out"=w381:errorcluster)  [unwired: 9 in]
            n147 = Merge Errors(w381, w379) -> (w380:errorcluster)
          }
          frame Default {
            # "'Default' case only runs if there is a message that isn't defined in any of the other cases.  Output a programming error."
            n148 = property class="Mod Admin"(reference=w385) -> ("Accessors:Module ID"=w384:i32)  [unwired: 1 in, 2 out]
            n149 = call "Module Name--constant.vi"("Module ID"=w384) -> ("Module Name"=w386:string)  [unwired: 10 in]
            n150 = xnode "Error Ring"("parameter 0"=w387, "parameter 1"=w386) -> ("error out"=w391:errorcluster)
            n151 = Merge Errors(w389, w391) -> (w390:errorcluster)
          }
        }
        n152 = call-dynamic "Delacor_lib_QMH_Error Handler - Message Handling Loop.vi"("error in"=w270, "Message Queue in"=w260) -> ("dup error in"=w267:errorcluster)  [unwired: 8 in, 1 out]
      }
      n153 = while {
        tunnel: w37 -> [w54]
        shift-right: [w51] -> _
        shift-left: -1 -> [w45]
        tunnel: w36 -> [w53]
        tunnel: [w50] -> w35
        tunnel: [w49] -> w34
        shift-right: [w47] -> _
        shift-left: w33 -> [w48]
        tunnel: w31 -> [w46]
        tunnel: w30 -> [w44]
        stop <- w52 stop-if-true
        n154 = event shown="[0] Timeout" {
          selector: w53 -> [_ _ _]
          dyn-events: [_ _ _] -> w49
          timeout: w45 -> [w58 _ _]
          tunnel: w54 -> [_ w90 w102]
          tunnel: [_ _ w99] -> w52
          tunnel: [w58 w79 w97] -> w51
          tunnel: [_ w88 w102] -> w50
          tunnel: w48 -> [w56 w86 w98]
          tunnel: [w56 w85 w98] -> w47
          tunnel: w46 -> [_ _ _]
          tunnel: w45 -> [_ w80 w97]
          tunnel: w44 -> [_ w78 w101]
          event Timeout {
            n155 = event-data() -> ()  [unwired: 1 in, 1 out]
            n156 = Unbundle By Name(w56) -> ("Active Signal"=w55:string[])
            n157 = for {
              tunnel: w55 -> [w59] mode=indexing
              tunnel: [w61] -> w57 mode=indexing
              n158 = call "Get Index and Type.vi"("Tag"=w59) -> ("Type"=w60:T11)  [unwired: 8 in, 2 out]
              n159 = case shown="\"Boolean\"" w60 {
                tunnel: [w63 w64 w67 w72] -> w61
                tunnel: w59 -> [w62 w66 w71 w77]
                frame "Array of Double" {
                  n160 = call-poly "Read.vi"("Tag Name"=w62) -> ("Value"=w63:dbl[])  [unwired: 9 in, 1 out]
                }
                frame "Double", Default {
                  n161 = call-poly "Read.vi"("Tag Name"=w66) -> ("Value"=w65:dbl)  [unwired: 9 in, 1 out]
                  n162 = Build Array(w65) -> (w64:dbl[])
                }
                frame "Single" {
                  n163 = call-poly "Read.vi"("Tag Name"=w71) -> ("Value"=w70:sgl)  [unwired: 9 in, 1 out]
                  n164 = Type Cast(type=0.0 ("Value"), x=w70) -> (*(type *) &x=w68:dbl)
                  n165 = Build Array(w68) -> (w67:dbl[])
                }
                frame "Boolean" {
                  n166 = call-poly "Read.vi"("Tag Name"=w77) -> ("Value"=w76:bool)  [unwired: 9 in, 1 out]
                  n167 = Select(t=i16 1 ("U8"), s=w76, f=i16 0 ("U8")) -> (s? t:f=w73:i16)
                  n168 = Build Array(w73) -> (w72:i16[])
                }
              }
            }
            "Analog Data" <- w57
          }
          event User Event {
            n169 = event-data() -> ("Timeout"=w81:i32, "Message Data"=w89:variant, "Module ID"=w83:i32)  [unwired: 1 in]
            n170 = call "Addressed to This Module.vi"("Module ID from Argument"=w83, "Module Admin"=w78) -> ("Addressed to this instance?"=w82:bool)  [unwired: 8 in, 1 out]
            n171 = Variant To Data(error in=w90, type=string[] [], Variant=w89) -> (data=w84:string[], error out=w88:errorcluster)
            n172 = case shown="True" w82 {
              tunnel: w86 -> [w91 w96]
              tunnel: [w91 w95] -> w85
              tunnel: w84 -> [_ w94]
              tunnel: w83 -> [_ _]
              tunnel: w81 -> [_ w93]
              tunnel: w80 -> [w92 _]
              tunnel: [w92 w93] -> w79
              frame False {
              }
              frame True {
                n173 = Bundle By Name(cluster=w96, "Active Signal"=w94) -> (w95:T10)
              }
            }
          }
          event User Event {
            n174 = event-data() -> ("Module ID"=w100:i32)  [unwired: 1 in]
            n175 = call "Addressed to This Module.vi"("Module ID from Argument"=w100, "Module Admin"=w101) -> ("Addressed to this instance?"=w99:bool)  [unwired: 8 in, 1 out]
          }
        }
      }
    }
    frame Error {
      n176 = call "Synchronize Caller Events.vi"("Module Admin"=w406) -> ("Module Admin out"=w405:refnum<class "Delacor_lib_QMH_Cloneable Module Admin.lvclass">)  [unwired: 9 in, 1 out]
      n177 = property class="Mod Admin"(reference=w405) -> ("Accessors:Module ID"=w404:i32)  [unwired: 1 in, 2 out]
      n178 = call-dynamic "Delacor_lib_QMH_Release Message Queue.vi"("error in"=w403, "Message Queue"=w401) -> ("error out"=w402:errorcluster)  [unwired: 9 in]
      n179 = call "Module Name--constant.vi"("Module ID"=w404) -> ("Module Name"=w409:string)  [unwired: 10 in]
      n180 = Format Into String(format string="An error occurred during initialization. %s is no longer running.", w409) -> (resulting string=w407:string)  [unwired: 2 in, 1 out]
      n181 = call "Error Reported.vi"("Additional Information"=w407, "Error"=w402, "Module ID"=w404) -> ()  [unwired: 8 in, 1 out]
    }
  }
  n182 = Merge Errors(w28, w27) -> (w29:errorcluster)
  n183 = call "Close Module.vi"("error in"=w29, "Wait for stop?"=w15, "Module Admin in"=w5) -> ("error out"=w25:errorcluster, "External Launch"=w14:bool, "Module Admin out"=w16:refnum<class "Delacor_lib_QMH_Cloneable Module Admin.lvclass">)  [unwired: 6 in]
  n184 = Unregister For Events(event registration refnum=w8, error in=w9) -> (error out=w6:errorcluster)
  n185 = Unregister For Events(event registration refnum=w20, error in=w25) -> (error out=w24:errorcluster)
  n186 = local write "Module Admin"(w16) -> ()
  n187 = case "External Launch?" shown="True" w14 {
    tunnel: w24 -> [_ w411]
    frame False {
    }
    frame True {
      n188 = case shown="No Error" w411 {
        frame No Error {
          n189 = invoke class="VI" method="FP.Close"() -> ()  [unwired: 3 in, 3 out]
        }
        frame Error {
          n190 = invoke class="VI" method="FP.Open"("Activate"=TRUE ("Activate?")) -> ()  [unwired: 4 in, 5 out]
        }
      }
    }
  }
  n191 = Merge Errors(w24, w6) -> (→"error out":errorcluster)
